vi "Indexing objective OG waveform_Bak.vi"(0 "Window size for layer index":dbl, 1 "OG start layer":dbl, 2 "OG end layer":dbl, 3 "Steps per Volume":dbl, 4 "OG repitation":dbl, 5 "Waveform":waveform(dbl), 6 "Objective 线性加速 时间 (s)":dbl, 7 "OG Z 线性加速 采样信息":cluster{"采样率":dbl, "采样数":dbl}, 9 "OG Z stack 刺激 steps 采样信息":cluster{"采样率":dbl, "采样数":dbl}, 10 "Objective volet 线性减速 时间 (s)":dbl, 11 "OG Z volet 线性减速 采样信息":cluster{"采样率":dbl, "采样数":dbl}, 12 "Objective 线性减速 时间 (s)":dbl, 13 "OG Z 线性减速 采样信息":cluster{"采样率":dbl, "采样数":dbl}) -> (14 "digital waveform":digitalwaveform(waveform))   [LabVIEW 2018]
uses:
  <vilib>/measure/mascope.llb/Transition Measurements 1 chan.vi
  <vilib>/Waveform/WDTOps.llb/WDT Append Waveforms DBL.vi
  <vilib>/Waveform/DWDTOps.llb/DWDT Analog to Digital.vi
  <vilib>/measure/NI_MABase.lvlib
  <vilib>/measure/NI_MAPro.lvlib
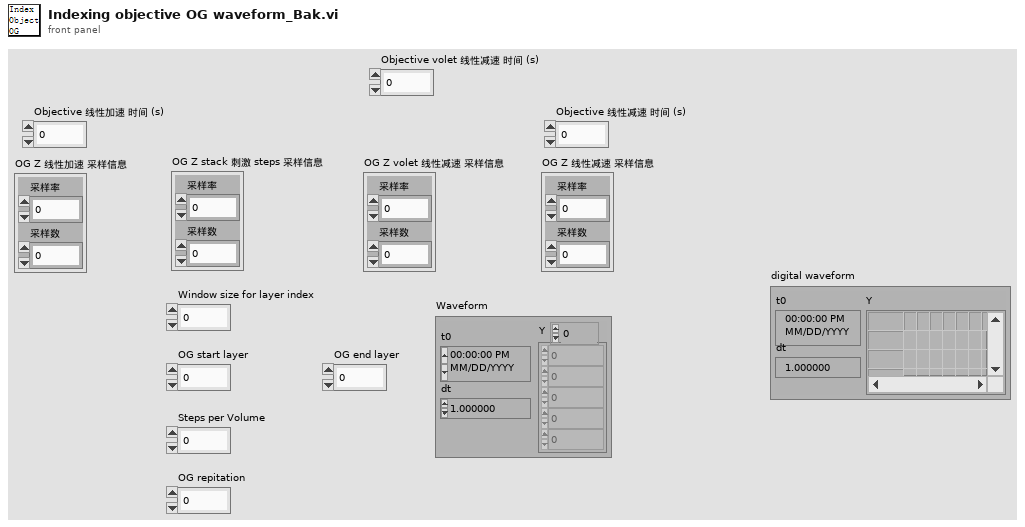
[diagram p1: front panel]
types:
  T1 = cluster{"high ref level":dbl, "mid ref level":dbl, "low ref level":dbl, "ref units":u16}
  T2 = cluster{"start time":dbl, "end time":dbl, "ref levels":cluster{"high ref level":dbl, "mid ref level":dbl, "low ref level":dbl, "ref units":u16}}
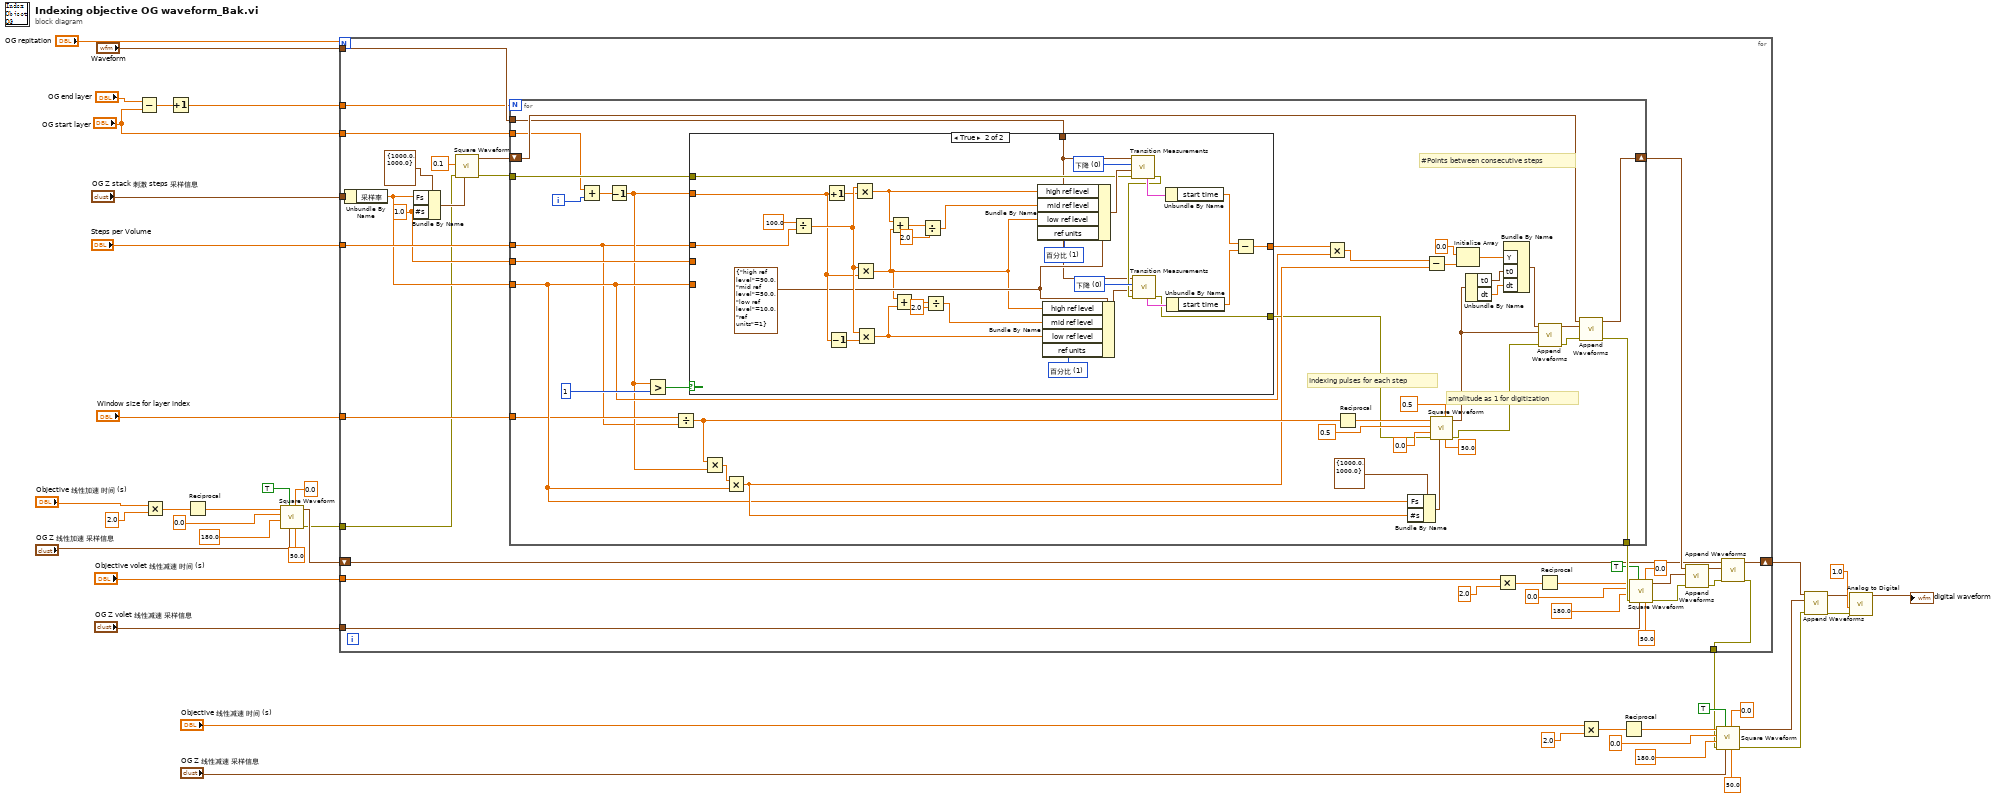
[diagram p0: block diagram]
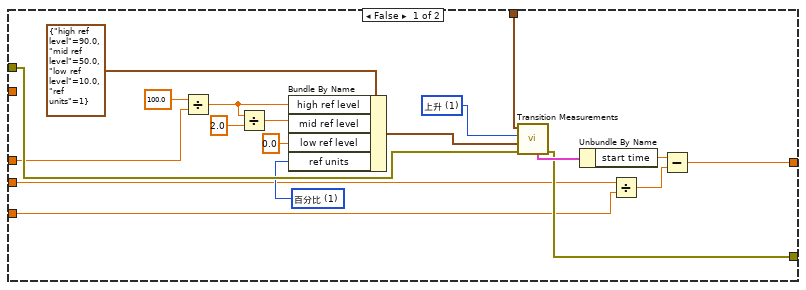
[diagram p2: hidden frame]
diagram:
  n1 = Subtract(x="OG end layer", y="OG start layer") -> (x-y=w32:dbl)
  n2 = Multiply(x="Objective 线性加速 时间 (s)", y=2.0) -> (x*y=w10:dbl)
  n3 = Increment(x=w32) -> (x+1=w31:dbl)
  n4 = Reciprocal(x=w10) -> (1/x=w11:dbl)
  n5 = call <vilib>:"Square Waveform.vi"("duty cycle (%)"=50.0, "offset"=0.0, "sampling info"="OG Z 线性加速 采样信息", "reset signal"=TRUE, "phase"=180.0, "amplitude"=0.0, "frequency"=w11) -> ("error out"=w3:errorcluster, "signal out"=w5:waveform(dbl))  [unwired: 3 in]
  n6 = for {
    N: "OG repitation" -> [_]
    tunnel: "Steps per Volume" -> [w74]
    tunnel: "Window size for layer index" -> [w73]
    tunnel: "OG Z stack 刺激 steps 采样信息" -> [w72]
    tunnel: "Waveform" -> [w71]
    tunnel: "OG Z volet 线性减速 采样信息" -> [w70]
    tunnel: "Objective volet 线性减速 时间 (s)" -> [w51]
    tunnel: w31 -> [w50]
    tunnel: "OG start layer" -> [w49]
    shift-right: [w48] -> w4
    shift-left: w5 -> [w45]
    tunnel: w3 -> [w44]
    tunnel: [w42] -> w2
    w68 = 1.0 ("#s")
    n7 = Unbundle By Name(w72) -> ("采样率"=w69:dbl)
    n8 = Bundle By Name(cluster=cluster{"Fs":dbl, "#s":dbl} {"Fs"=1000.0, "#s"=1000.0} ("sampling info"), "Fs"=w69, "#s"=w68) -> (w64:cluster{"Fs":dbl, "#s":dbl})
    n9 = call <vilib>:"Square Waveform.vi"("sampling info"=w64, "error in (no error)"=w44, "amplitude"=0.1) -> ("error out"=w67:errorcluster, "signal out"=w65:waveform(dbl))  [unwired: 7 in]
    n10 = for {
      N: w50 -> [_]
      shift-right: [w92] -> w46
      shift-left: w65 -> [w93]
      tunnel: [w88] -> w66
      tunnel: w67 -> [w87]
      tunnel: w68 -> [w81]
      tunnel: w69 -> [w86]
      tunnel: w71 -> [w82]
      tunnel: w74 -> [w75]
      tunnel: w73 -> [w80]
      tunnel: w49 -> [w76]
      i -> [w77]
      # "amplitude as 1 for digitization"
      # "Indexing pulses for each step"
      # "#Points between consecutive steps"
      n11 = Add(x=w76, y=w77) -> (x+y=w79:dbl)
      n12 = Decrement(x=w79) -> (x-1=w78:dbl)
      n13 = Greater?(x=w78, y=1) -> (0:w102:bool)
      n14 = Divide(x=w80, y=w75) -> (x/y=w107:dbl)
      n15 = case shown="True" w102 {
        tunnel: w82 -> [w131 w133]
        tunnel: w78 -> [_ w156]
        tunnel: [w117 w149] -> w100
        tunnel: [w123 w147] -> w91
        tunnel: w87 -> [w124 w146]
        tunnel: w81 -> [w115 _]
        tunnel: w86 -> [w114 _]
        tunnel: w75 -> [w113 w132]
        frame False {
          w122 = u16 1 items=["绝对", "百分比"] ("ref units")
          w130 = u16 1 items=["下降", "上升"] ("polarity (rising)")
          n16 = Divide(x=100.0, y=w113) -> (x/y=w120:dbl)
          n17 = Divide(x=w120, y=2.0) -> (x/y=w121:dbl)
          n18 = Bundle By Name(cluster=T1 {"high ref level"=90.0, "mid ref level"=50.0, "low ref level"=10.0, "ref units"=1} ("reference levels 2"), "high ref level"=w120, "mid ref level"=w121, "low ref level"=0.0, "ref units"=w122) -> (w128:T1)
          n19 = call-poly <vilib>:"Transition Measurements.vi"("error in (no error)"=w124, "reference levels"=w128, "polarity (rising)"=w130, "signal in"=w131) -> ("error out"=w123:errorcluster, "measurement info"=w125:T2)  [unwired: 2 in, 4 out]
          n20 = Unbundle By Name(w125) -> ("start time"=w118:dbl)
          n21 = Divide(x=w115, y=w114) -> (x/y=w116:dbl)
          n22 = Subtract(x=w118, y=w116) -> (x-y=w117:dbl)
        }
        frame True {
          w144 = u16 1 items=["绝对", "百分比"] ("ref units")
          w145 = u16 1 items=["绝对", "百分比"] ("ref units 2")
          w152 = T1 {"high ref level"=90.0, "mid ref level"=50.0, "low ref level"=10.0, "ref units"=1} ("reference levels")
          w160 = u16 0 items=["下降", "上升"] ("polarity (rising)")
          w162 = u16 0 items=["下降", "上升"] ("polarity (rising)")
          n23 = Divide(x=100.0, y=w132) -> (x/y=w157:dbl)
          n24 = Increment(x=w156) -> (x+1=w155:dbl)
          n25 = Decrement(x=w156) -> (x-1=w154:dbl)
          n26 = Multiply(x=w157, y=w155) -> (x*y=w136:dbl)
          n27 = Multiply(x=w157, y=w156) -> (x*y=w134:dbl)
          n28 = Multiply(x=w157, y=w154) -> (x*y=w135:dbl)
          n29 = Add(x=w136, y=w134) -> (x+y=w142:dbl)
          n30 = Add(x=w134, y=w135) -> (x+y=w140:dbl)
          n31 = Divide(x=w142, y=2.0) -> (x/y=w141:dbl)
          n32 = Divide(x=w140, y=2.0) -> (x/y=w139:dbl)
          n33 = Bundle By Name(cluster=w152, "high ref level"=w136, "mid ref level"=w141, "low ref level"=w134, "ref units"=w144) -> (w153:T1)
          n34 = Bundle By Name(cluster=w152, "high ref level"=w134, "mid ref level"=w139, "low ref level"=w135, "ref units"=w145) -> (w143:T1)
          n35 = call-poly <vilib>:"Transition Measurements.vi"("error in (no error)"=w146, "reference levels"=w153, "polarity (rising)"=w160, "signal in"=w133) -> ("error out"=w148:errorcluster, "measurement info"=w158:T2)  [unwired: 2 in, 4 out]
          n36 = call-poly <vilib>:"Transition Measurements.vi"("error in (no error)"=w148, "reference levels"=w143, "polarity (rising)"=w162, "signal in"=w133) -> ("error out"=w147:errorcluster, "measurement info"=w161:T2)  [unwired: 2 in, 4 out]
          n37 = Unbundle By Name(w158) -> ("start time"=w151:dbl)
          n38 = Unbundle By Name(w161) -> ("start time"=w150:dbl)
          n39 = Subtract(x=w151, y=w150) -> (x-y=w149:dbl)
        }
      }
      n40 = Multiply(x=w107, y=w78) -> (x*y=w106:dbl)
      n41 = Multiply(x=w106, y=w86) -> (x*y=w99:dbl)
      n42 = Multiply(x=w100, y=w86) -> (x*y=w101:dbl)
      n43 = Reciprocal(x=w107) -> (1/x=w112:dbl)
      n44 = Bundle By Name(cluster=cluster{"Fs":dbl, "#s":dbl} {"Fs"=1000.0, "#s"=1000.0} ("sampling info"), "Fs"=w86, "#s"=w99) -> (w104:cluster{"Fs":dbl, "#s":dbl})
      n45 = Subtract(x=w101, y=w99) -> (x-y=w98:dbl)
      n46 = call <vilib>:"Square Waveform.vi"("duty cycle (%)"=50.0, "offset"=0.5, "sampling info"=w104, "error in (no error)"=w91, "phase"=0.0, "amplitude"=0.5, "frequency"=w112) -> ("error out"=w90:errorcluster, "signal out"=w83:waveform(dbl))  [unwired: 3 in]
      n47 = Initialize Array(0.0 ("元素"), w98) -> (w96:dbl[])
      n48 = Unbundle By Name(w83) -> ("t0"=w85:timestamp, "dt"=w84:dbl)
      n49 = Bundle By Name("Y"=w96, "t0"=w85, "dt"=w84) -> (w95:waveform(dbl))  [unwired: 1 in]
      n50 = call-poly <vilib>:"Append Waveforms.vi"("error in (no error)"=w90, "waveform B"=w83, "waveform A"=w95) -> ("error out"=w89:errorcluster, "waveform out"=w94:waveform(dbl))  [unwired: 7 in]
      n51 = call-poly <vilib>:"Append Waveforms.vi"("error in (no error)"=w89, "waveform B"=w94, "waveform A"=w93) -> ("error out"=w88:errorcluster, "waveform out"=w92:waveform(dbl))  [unwired: 7 in]
    }
    n52 = Multiply(x=w51, y=2.0) -> (x*y=w53:dbl)
    n53 = Reciprocal(x=w53) -> (1/x=w54:dbl)
    n54 = call <vilib>:"Square Waveform.vi"("duty cycle (%)"=50.0, "offset"=0.0, "sampling info"=w70, "reset signal"=TRUE, "error in (no error)"=w66, "phase"=180.0, "amplitude"=0.0, "frequency"=w54) -> ("error out"=w59:errorcluster, "signal out"=w58:waveform(dbl))  [unwired: 2 in]
    n55 = call-poly <vilib>:"Append Waveforms.vi"("error in (no error)"=w59, "waveform B"=w58, "waveform A"=w46) -> ("error out"=w43:errorcluster, "waveform out"=w47:waveform(dbl))  [unwired: 7 in]
    n56 = call-poly <vilib>:"Append Waveforms.vi"("error in (no error)"=w43, "waveform B"=w47, "waveform A"=w45) -> ("error out"=w42:errorcluster, "waveform out"=w48:waveform(dbl))  [unwired: 7 in]
  }
  n57 = Multiply(x="Objective 线性减速 时间 (s)", y=2.0) -> (x*y=w23:dbl)
  n58 = Reciprocal(x=w23) -> (1/x=w24:dbl)
  n59 = call <vilib>:"Square Waveform.vi"("duty cycle (%)"=50.0, "offset"=0.0, "sampling info"="OG Z 线性减速 采样信息", "reset signal"=TRUE, "error in (no error)"=w2, "phase"=180.0, "amplitude"=0.0, "frequency"=w24) -> ("error out"=w18:errorcluster, "signal out"=w17:waveform(dbl))  [unwired: 2 in]
  n60 = call-poly <vilib>:"Append Waveforms.vi"("error in (no error)"=w18, "waveform B"=w17, "waveform A"=w4) -> ("error out"=w19:errorcluster, "waveform out"=w1:waveform(dbl))  [unwired: 7 in]
  n61 = call-poly <vilib>:"Analog to Digital.vi"("error in (no error)"=w19, "full-scale range (pk-pk)"=1.0, "analog waveform"=w1) -> ("digital waveform"=→"digital waveform":digitalwaveform)  [unwired: 5 in, 3 out]
